vi "Execute Convert Enum.vi"(6 "Mouse Position":T1 caption="鼠标位置", 8 "User VI Ref":refnum<vi> caption="用户VI引用", 9 "Menu Item Tag Suffix":string caption="菜单项标签后缀", 10 "Remaining Items":refnum<vi>[](array[refnum]) caption="剩余项", 11 "Affected Items":T2 caption="受影响的项") -> (0 "Fail transaction?":bool caption="操作失败？")   [LabVIEW 2020]
doc: "该VI属于修改LabVIEW快捷菜单部分。这是用户选择快捷菜单时调用的执行VI。该VI执行选中菜单项的操作。"
uses:
  Convert Enum.ctl
  <vilib>/Utility/miscctls.llb/LVPositionTypeDef.ctl
panel:
  # "除“受影响的项”之外，前面板上的其他所有控件都已锁定，以防被意外编辑。修改控件名称或类型，而不是“受影响的项”簇的元素将使VI无法作为菜单插件使用。\n\n请参考每个控件的即时帮助了解其用法。"
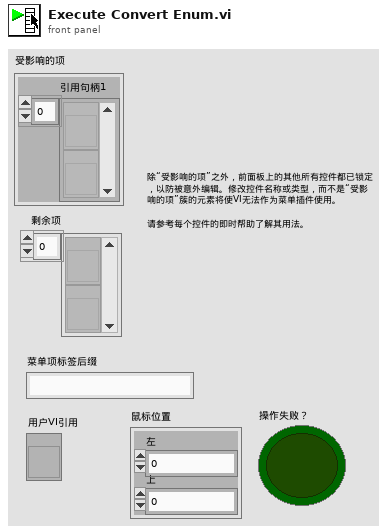
[diagram p1: front panel]
types:
  T1 = typedef "LVPositionTypeDef.ctl" = cluster{"Left":i32, "Top":i32}
  T2 = typedef "Convert Enum.ctl" = cluster{"Refnums 1":refnum<vi>[]}
  T3 = typedef "LVStringsAndValuesArrayTypeDef.ctl" = cluster{"String":string, "Value":ext}[]
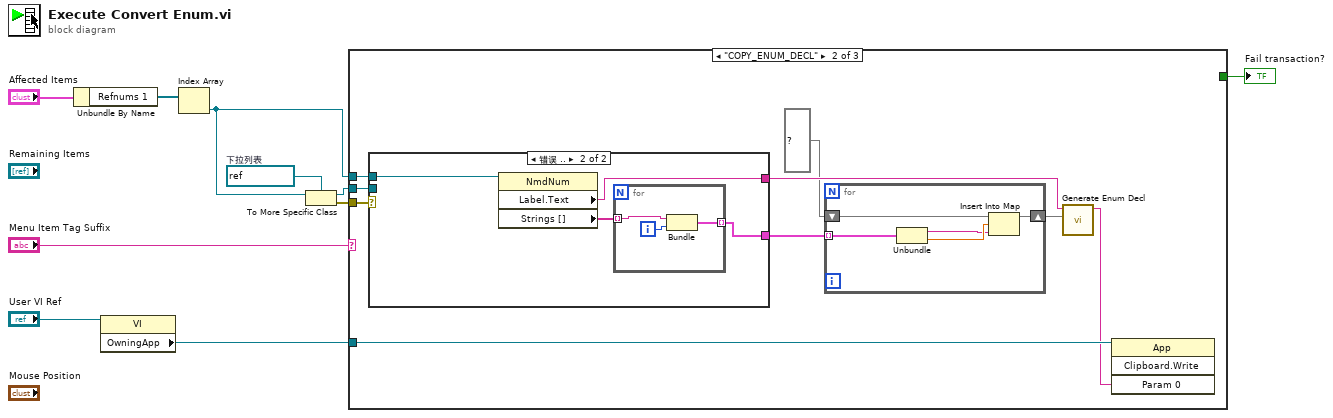
[diagram p0: block diagram]
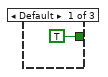
[diagram p2: hidden frame]
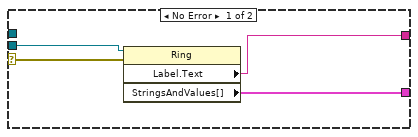
[diagram p3: hidden frame]
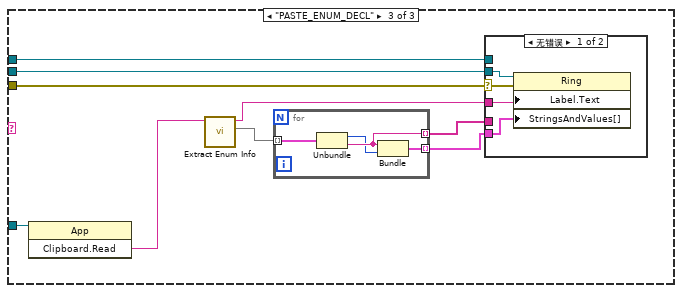
[diagram p4: hidden frame]
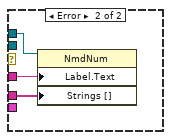
[diagram p5: hidden frame]
diagram:
  w6 = refnum<vi> refnum  # 下拉列表
  n1 = Unbundle By Name("Affected Items") -> ("Refnums 1"=w9:refnum<vi>[])
  n2 = property class="VI"(reference="User VI Ref") -> ("OwningApp"=w7:refnum<vi>)  [unwired: 1 in, 2 out]
  n3 = Index Array(array=w9) -> (element=w3:refnum<vi>)  [unwired: 1 in]
  n4 = To More Specific Class(target class=w6, reference=w3) -> (specific class reference=w4:refnum<vi>, error out=w5:errorcluster)  [unwired: 1 in]
  n5 = case shown="\"COPY_ENUM_DECL\"" "Menu Item Tag Suffix" {
    tunnel: w7 -> [_ w14 w45]
    tunnel: w5 -> [_ w20 w43]
    tunnel: w4 -> [_ w19 w42]
    tunnel: w3 -> [_ w12 w38]
    tunnel: [TRUE ("Fail transaction?") _ _] -> w1
    frame Default {
    }
    frame "COPY_ENUM_DECL" {
      n6 = case shown="错误 .." w20 {
        selector: w20 -> [w29 _]
        tunnel: w19 -> [w28 _]
        tunnel: [w27 w33] -> w18
        tunnel: [w26 w31] -> w15
        tunnel: w12 -> [_ w30]
        frame No Error {
          n7 = property class="Ring"(reference=w28, error in=w29) -> ("Label.Text"=w27:string, "StringsAndValues[]"=w26:T3)  [unwired: 2 out]
        }
        frame Error {
          n8 = property class="NmdNum"(reference=w30) -> ("Label.Text"=w33:string, "Strings []"=w32:string[])  [unwired: 1 in, 2 out]
          n9 = for {
            tunnel: w32 -> [w36] mode=indexing
            tunnel: [w34] -> w31 mode=indexing
            i -> [w35]
            n10 = Bundle(w36, w35) -> (w34:cluster{string, i32})  [unwired: 1 in]
          }
        }
      }
      n11 = for {
        shift-right: [w25] -> w17
        shift-left: map{u32, string} {} ("枚举列表") -> [w24]
        tunnel: w15 -> [w23] mode=indexing
        n12 = Unbundle(w23) -> ("String"=w21:string, "Value"=w22:ext)
        n13 = Insert Into Map(map in=w24, key=w22, value=w21) -> (map out=w25:map{u32, string})  [unwired: 2 out]
      }
      n14 = call "Generate Enum Decl.vi"("枚举列表"=w17, "枚举名称"=w18) -> ("枚举声明"=w13:string)  [unwired: 9 in]
      n15 = invoke class="App" method="Clipboard.Write"(reference=w14, "Param 0"=w13) -> ()  [unwired: 2 in, 4 out]
    }
    frame "PASTE_ENUM_DECL" {
      n16 = invoke class="App" method="Clipboard.Read"(reference=w45) -> ("Read Clipbrd"=w44:string)  [unwired: 2 in, 2 out]
      n17 = call "Extract Enum Info.vi"("enum"=w44) -> ("映射表"=w40:map{u32, string}, "枚举名称"=w41:string)  [unwired: 9 in]
      n18 = for {
        tunnel: w40 -> [w49] mode=indexing
        tunnel: [w48] -> w39 mode=indexing
        tunnel: [w46] -> w37 mode=indexing
        n19 = Unbundle(w49) -> ("key"=w47:u32, "value"=w48:string)
        n20 = Bundle("value"=w48, "key"=w47) -> (w46:cluster{"value":string, "key":u32})  [unwired: 1 in]
      }
      n21 = case shown="无错误" w43 {
        selector: w43 -> [w52 _]
        tunnel: w42 -> [w53 _]
        tunnel: w41 -> [w51 w54]
        tunnel: w39 -> [_ w55]
        tunnel: w38 -> [_ w56]
        tunnel: w37 -> [w50 _]
        frame No Error {
          n22 = property class="Ring"(reference=w53, error in=w52, "Label.Text"=w51, "StringsAndValues[]"=w50) -> ()  [unwired: 2 out]
        }
        frame Error {
          n23 = property class="NmdNum"(reference=w56, "Label.Text"=w54, "Strings []"=w55) -> ()  [unwired: 1 in, 2 out]
        }
      }
    }
  }
  "Fail transaction?" <- w1
